vi "Cascade S-parameters.vi"(8 "error in (no error)":errorcluster, 10 "S-par array 2 in":cdb[][](array[numeric]), 11 "S-par array 1 in":cdb[][](array[numeric])) -> (0 "error out":errorcluster, 3 "Cascaded S-par array out":cdb[][](array[numeric]))   [LabVIEW 2023, in "NI_HFNetworkAnalysis.lvlib"]
doc: "Cascades two networks defined by their S-parameters.\n\nTransformation assumes that the even ports of network 1 are connected to the odd ports of network 2.\n\nInput and output S-parameter array rows are defined as \n<b>(S11,S12,S13,S14,...,S21,S22,S23,S24,...,S31,S32,S33,S34,...,S41,S42,S43,S44,...)</b>\n\n<b>Known Limitations</b>\nTransformation supports only 2n-port networks."
uses:
  NI_HFNetworkAnalysis.lvlib
  <vilib>/Analysis/baseanly.llb/Complex A x B.vi
  <vilib>/Analysis/Matrix/Numeric/Conversions/Array To Matrix - CA2.vi
  <vilib>/Analysis/Matrix/NI_Matrix.lvlib
  <vilib>/Analysis/NI_AALBase.lvlib
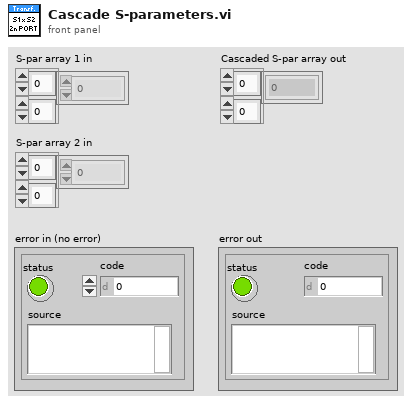
[diagram p1: front panel]
types:
  T1 = typedef "NI_Matrix.lvlib/ComplexMatrix.ctl" = cdb[][]
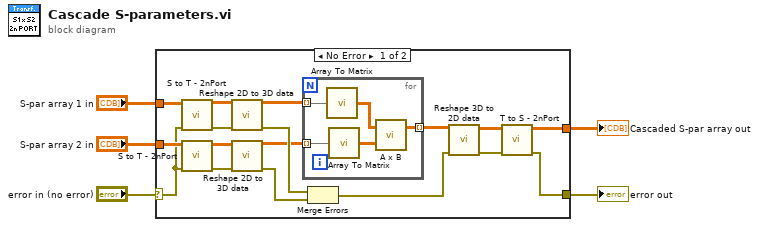
[diagram p0: block diagram]
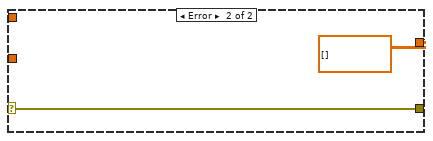
[diagram p2: hidden frame]
diagram:
  n1 = case shown="No Error" "error in (no error)" {
    selector: "error in (no error)" -> [w12 w29]
    tunnel: [w8 w29] -> w5
    tunnel: [w7 cdb[][] [] ("Parameters Out (2D)")] -> w4
    tunnel: "S-par array 2 in" -> [w22 _]
    tunnel: "S-par array 1 in" -> [w21 _]
    frame No Error {
      n2 = call "S to T - 2nPort.vi"("error in (no error)"=w12, "S-par Array In"=w21) -> ("error out"=w18:errorcluster, "T-par Array Out"=w19:cdb[][])  [unwired: 8 in]
      n3 = call "S to T - 2nPort.vi"("error in (no error)"=w12, "S-par Array In"=w22) -> ("error out"=w17:errorcluster, "T-par Array Out"=w20:cdb[][])  [unwired: 8 in]
      n4 = call "Reshape 2D to 3D data.vi"("Parameters In (2D)"=w19, "Error In"=w18) -> ("Parameters Out (3D)"=w16:cdb[][][], "Error Out"=w10:errorcluster)  [unwired: 12 in]
      n5 = call "Reshape 2D to 3D data.vi"("Parameters In (2D)"=w20, "Error In"=w17) -> ("Parameters Out (3D)"=w6:cdb[][][], "Error Out"=w11:errorcluster)  [unwired: 12 in]
      n6 = for {
        tunnel: w16 -> [w27] mode=indexing
        tunnel: w6 -> [w26] mode=indexing
        tunnel: [w23] -> w15 mode=indexing
        n7 = call-poly <vilib>:"Array To Matrix.vi"("Complex 2D Array"=w27) -> ("Complex Matrix"=w25:T1)
        n8 = call-poly <vilib>:"Array To Matrix.vi"("Complex 2D Array"=w26) -> ("Complex Matrix"=w24:T1)
        n9 = call-poly <vilib>:"A x B.vi"("B"=w24, "A"=w25) -> ("A x B"=w23:T1)  [unwired: 1 out]
      }
      n10 = Merge Errors(w10, w11) -> (w9:errorcluster)
      n11 = call "Reshape 3D to 2D data.vi"("Parameters In (3D)"=w15, "Error In"=w9) -> ("Parameters Out (2D)"=w14:cdb[][], "Error Out"=w13:errorcluster)  [unwired: 12 in]
      n12 = call "T to S - 2nPort.vi"("error in (no error)"=w13, "T-par Array In"=w14) -> ("error out"=w8:errorcluster, "S-par Array Out"=w7:cdb[][])  [unwired: 8 in]
    }
    frame Error {
    }
  }
  "error out" <- w5
  "Cascaded S-par array out" <- w4
